vi "Pause Resume OPC UA.vi"(8 "error in (no error)":errorcluster, 10 "Pause/Resume":bool, 11 "Panel in":refnum<class "Panel.lvclass">) -> (0 "error out":errorcluster, 3 "Panel out":refnum<class "Panel.lvclass">)   [LabVIEW 2021, in "Panel.lvlib" / "Panel.lvclass"]
uses:
  Panel.lvclass
  C:/Program Files/National Instruments/LabVIEW 2021/vi.lib/ActorFramework/Actor/Actor.lvclass
  <vilib>/ActorFramework/Actor/Actor.lvclass/Actor.ctl
  Panel.lvclass/Panel.ctl
  Station State Interface/Station Status Messages/Update Enable Msg/Update Enable Msg.lvclass/Update Enable Msg.ctl
  <vilib>/ActorFramework/Message Enqueuer/Message Enqueuer.lvclass/Message Enqueuer.ctl
  <vilib>/ActorFramework/Message Enqueuer/Enqueue.vi
  Station State Interface/Station Status Messages/Update Enable Msg/Update Enable Msg.lvclass
  C:/Program Files/National Instruments/LabVIEW 2021/vi.lib/ActorFramework/Message/Message.lvclass
  <vilib>/ActorFramework/Message Priority Queue/Priority Enqueue.vi
  <vilib>/ActorFramework/Actor/Actor.lvclass
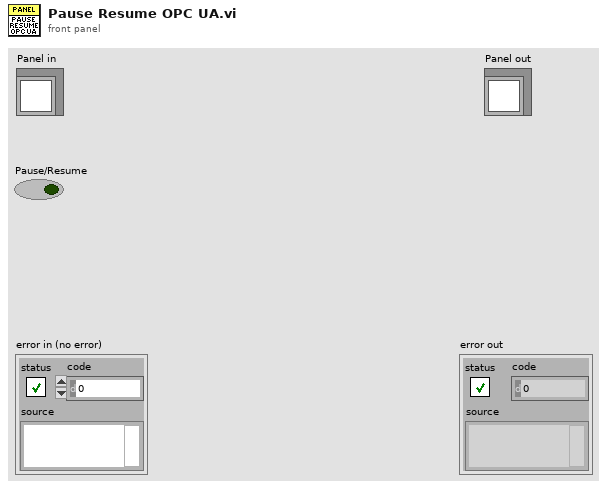
[diagram p1: front panel]
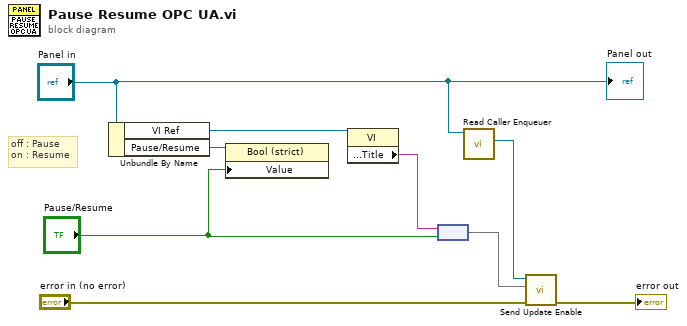
[diagram p0: block diagram]
diagram:
  # "off : Pause\non : Resume"
  n1 = Unbundle By Name("Panel in") -> ("VI Ref"=w4:refnum<vi>, "Pause/Resume"=w9:refnum<vi>)
  n2 = property class="Bool (strict)"(reference=w9, "Value"="Pause/Resume") -> ()  [unwired: 1 in, 2 out]
  n3 = property class="VI"(reference=w4) -> ("Front Panel.Title"=w3:string)  [unwired: 1 in, 2 out]
  n4 = node(w3, "Pause/Resume") -> (w8:map{string, bool})
  n5 = call <vilib>:"Read Caller Enqueuer.vi"("Actor"="Panel in") -> ("Caller Enqueuer"=w1:refnum<class "Message Enqueuer.lvclass">)  [unwired: 10 in]
  n6 = call "Send Update Enable.vi"("error in (no error)"="error in (no error)", "Station Status"=w8, "Message Enqueuer"=w1) -> ("error out"=→"error out":errorcluster)  [unwired: 7 in, 1 out]
  "Panel out" <- "Panel in"
